vi "To String.vi"(8 "error in":errorcluster, 11 "value":variant) -> (0 "error out":errorcluster, 2 "string":string, 3 "value dup":variant)   [LabVIEW 2020, in "Value.lvlib"]
uses:
  Value.lvlib
  Display.ctl
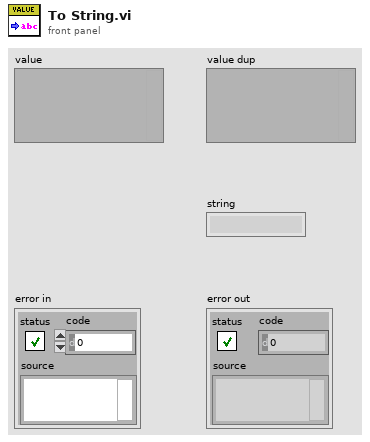
[diagram p1: front panel]
types:
  T1 = typedef "Value.lvlib/Display.ctl" = cluster{"Limit Low":dbl, "Limit High":dbl, "Description":string, "Units":string, "Precision":i32, "Form":enum32{"Default", "String", "Binary", "Decimal", "Hex", "Exponential", "Engineering"}}
  T2 = typedef "Value.lvlib/Type Code.ctl" = enum8{"Null", "Bool", "BoolA", "Int8", "Int8A", "Int16", "Int16A", "Int32", "Int32A", "Int64", "Int64A", "UInt8", "UInt8A", "UInt16", "UInt16A", "UInt32", "UInt32A", "UInt64", "UInt64A", "Float32", "Float32A", "Float64", "Float64A", "String", "StringA", "Struct", "StructA", "Union", "UnionA", "Any", "AnyA"}
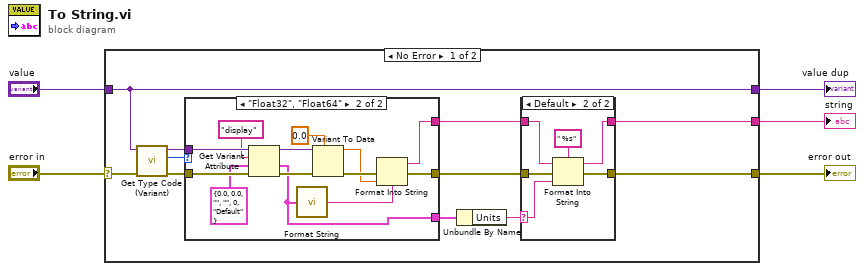
[diagram p0: block diagram]
diagram:
  n1 = case shown="No Error" "error in" {
    selector: "error in" -> [w13 w40]
    tunnel: [w8 w40] -> w5
    tunnel: "value" -> [w12 w39]
    tunnel: [w12 w39] -> w2
    tunnel: [w6 _] -> w1
    frame No Error {
      n2 = call "Get Type Code (Variant).vi"("error in (no error)"=w13, "value"=w12) -> ("error out"=w16:errorcluster, "type code"=w15:T2, "value dup"=w14:variant)  [unwired: 5 in]
      n3 = case shown="\"Float32\", \"Float64\"" w15 {
        tunnel: w16 -> [w25 w31]
        tunnel: w14 -> [_ w32]
        tunnel: [w25 w36] -> w9
        tunnel: [_ w27] -> w7
        tunnel: [_ w26] -> w11
        frame Default {
        }
        frame "Float32", "Float64" {
          n4 = Get Variant Attribute(Variant=w32, name="display", default value (empty Variant)=T1 {"Limit Low"=0.0, "Limit High"=0.0, "Description"="", "Units"="", "Precision"=0, "Form"=enum."Default"} ("Display"), error in=w31) -> (duplicate Variant=w33:variant, value=w26:T1, error out=w34:errorcluster)  [unwired: 1 out]
          n5 = call "Format String.vi"("Display"=w26) -> ("format"=w28:string)
          n6 = Variant To Data(error in=w34, type=0.0, Variant=w33) -> (data=w35:dbl, error out=w37:errorcluster)
          n7 = Format Into String(format string=w28, error in=w37, w35) -> (resulting string=w27:string, error out=w36:errorcluster)  [unwired: 1 in]
        }
      }
      n8 = Unbundle By Name(w11) -> ("Units"=w10:string)
      n9 = case shown="Default" w10 {
        selector: w10 -> [_ w19]
        tunnel: [w18 w23] -> w8
        tunnel: w9 -> [w18 w24]
        tunnel: w7 -> [w17 w21]
        tunnel: [w17 w20] -> w6
        frame "" {
        }
        frame Default {
          n10 = Format Into String(format string=" %s", initial string=w21, error in=w24, w19) -> (resulting string=w20:string, error out=w23:errorcluster)
        }
      }
    }
    frame Error {
    }
  }
  "error out" <- w5
  "string" <- w1
  "value dup" <- w2
